vi "STFT.vi"() -> ()   [LabVIEW 2023]
uses:
  <vilib>/Analysis/4window.llb/windowTd.ctl
  <vilib>/express/express analysis/Spectral/Block/exnSpectralBlock spectral measurements RMS poly.vi
  <vilib>/express/express analysis/Spectral/Block/exnSpectralBlock spectral measurements RMS array WFM.vi
  <vilib>/express/express analysis/Spectral/XNode/ExpressSpectralMeasurementsBlockNode.xnode
  <vilib>/gmath/NI_Gmath.lvlib
  <vilib>/Analysis/NI_AALPro.lvlib
panel:
  out "data":waveform(dbl)[](graph)
  out "STFT Spectrogram":dbl[][](graph)
  in  "window info":cluster{"type":T1, "length":i32}={"type"=1, "length"=1024} {"type" items=["Rectangle"=0, "Hanning"=1, "Hamming"=2, "Blackman-Harris"=3, "Exact Blackman"=4, "Blackman"=5, "Flat Top"=6, "4 Term B-Harris "=7, "7 Term B-Harris"=8, "Low Sidelobe"=9, "Blackman Nuttall"=11, "Triangle"=30, "Bartlett-Hanning"=31, "Bohman"=32, "Parzen"=33, "Welch"=34, "Kaiser"=60, "Dolph-Chebyshev"=61, "Gaussian"=62]}
  in  "time-freq sampling info":cluster{"time steps":i32, "frequency bins":i32}={"time steps"=10, "frequency bins"=1024}
  out "S(f)":cluster{"f0":dbl, "df":dbl, "magnitude":dbl[]}[](graph)
  in  "path":path
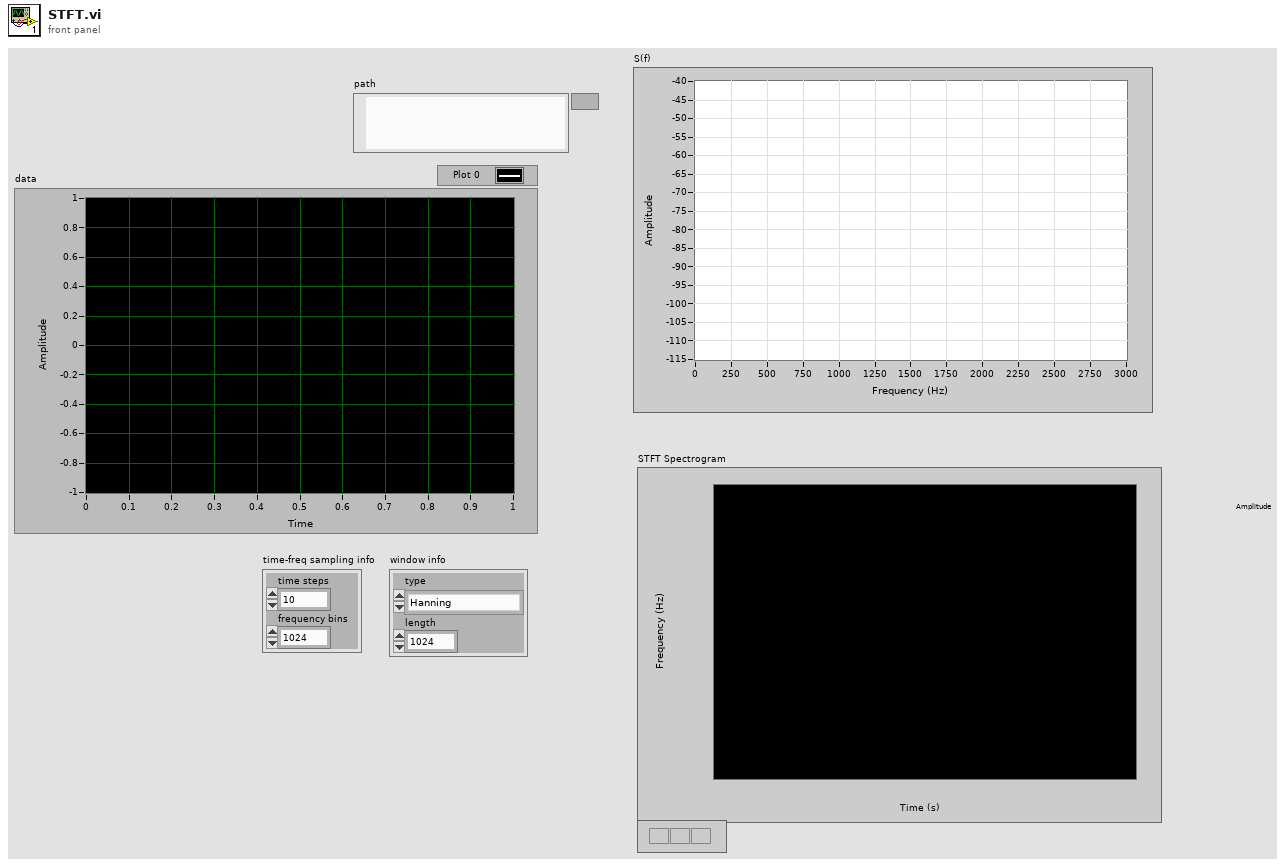
[diagram p1: front panel]
types:
  T1 = typedef "NI_AALPro.lvlib/windowTd.ctl" = u32
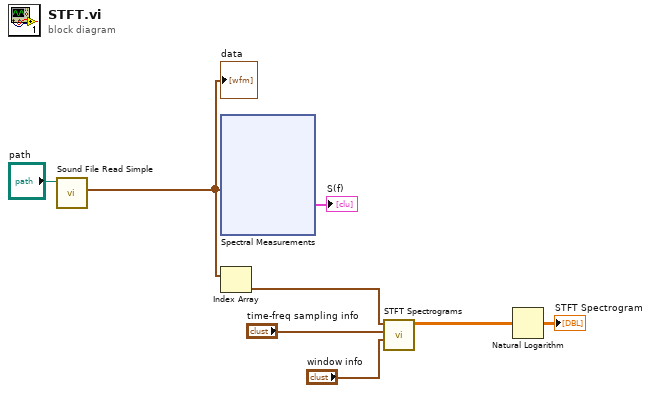
[diagram p0: block diagram]
diagram:
  n1 = call <vilib>:"Sound File Read Simple.vi"("path"="path") -> ("data"=w2:waveform(dbl)[])  [unwired: 7 in, 3 out]
  "data" <- w2
  n2 = xnode "Spectral Measurements"("Signals"=w2) -> ("FFT - (RMS)"=→"S(f)":cluster{"f0":dbl, "df":dbl, "magnitude":dbl[]}[])  [unwired: 1 in, 2 out]
  n3 = Index Array "Index Array"(array=w2) -> (element=w1:waveform(dbl))  [unwired: 1 in]
  n4 = call <vilib>:"STFT Spectrograms.vi"("window info"="window info", "time-freq sampling info"="time-freq sampling info", "X"=w1) -> ("STFT Spectrogram {X}"=w6:dbl[][])  [unwired: 7 in, 1 out]
  n5 = Natural Logarithm(1:w6) -> (0:→"STFT Spectrogram":dbl[][])
